vi "EditCut.vi"() -> (3 "Image out":refnum<class "Image.lvclass">)   [LabVIEW 2021, in "Menu.lvlib" / "Menu.lvclass"]
uses:
  Menu.lvclass
  Menu.lvclass/Menu.ctl
  Picture2D/src/Picture/Image.lvclass
  Picture2D/src/Point/Point.lvclass
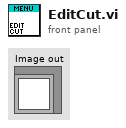
[diagram p1: front panel]
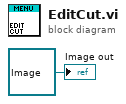
[diagram p0: block diagram]
diagram:
  "Image out" <- refnum<class "Image.lvclass"> refnum ("Image out")
